vi "Convert filetype to Is LabVIEW document.vi"(4 "file type":T1) -> (1 "Is LabVIEW document?":bool)   [LabVIEW 2019, in "NI_FileType.lvlib"]
doc: "Returns TRUE if this file type could be opened by LabVIEW. It uses the same criteria as the File >> Open dialog."
uses:
  NI_FileType.lvlib
  FT_FileTypes.ctl
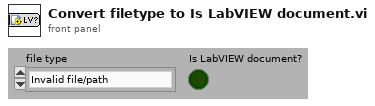
[diagram p1: front panel]
types:
  T1 = typedef "NI_FileType.lvlib/FT_FileTypes.ctl" = enum32{"Invalid file/path", "Unknown type", "Instrument", "Control", "Polymorphic VI", "Project", "Library", "LVClass", "XControl", "XNode", "CIN", "Run-time menu", "Palette menu", "LLB", "Shortcut", "Directory", "Class Private Data Control", "Statechart", "MathScript .m file", "Ladder Diagram", "LVLibp"}
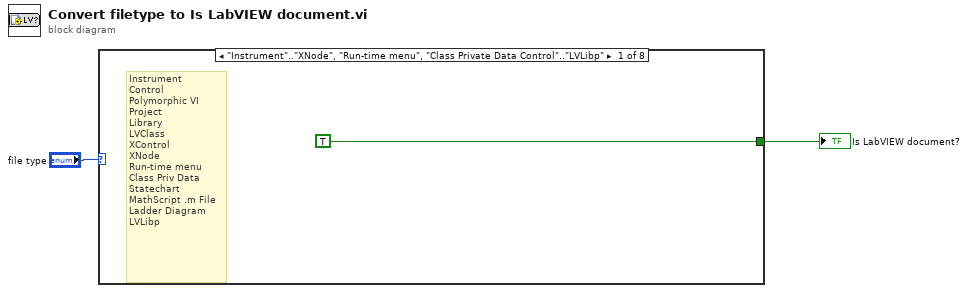
[diagram p0: block diagram]
diagram:
  n1 = case shown="\"Instrument\"..\"XNode\", \"Run-time menu\", \"Class Private Data Control\"..\"LVLibp\"" "file type" {
    tunnel: [TRUE _ _ _ _ _ _ _] -> w1
    frame "Instrument".."XNode", "Run-time menu", "Class Private Data Control".."LVLibp" {
      # "Instrument\nControl\nPolymorphic VI\nProject\nLibrary\nLVClass\nXControl\nXNode\nRun-time menu\nClass Priv Data\nStatechart\nMathScript .m File\nLadder Diagram\nLVLibp"
    }
    frame "CIN" {
    }
    frame "Palette menu" {
    }
    frame "LLB" {
    }
    frame "Shortcut" {
    }
    frame "Directory" {
    }
    frame "Unknown type" {
    }
    frame "Invalid file/path" {
    }
  }
  "Is LabVIEW document?" <- w1
